vi "LAKESHORE_10_01_2023_R_VS_T_DEMO_1.vi"() -> ()   [LabVIEW 2020]
panel:
  out "Resistance":dbl
  out "Temperature":dbl
  in  "Channel":T1(ring)
  in  "VISA resource name":refnum<visa-resource-name>
  # "LAKE SHORE 372"
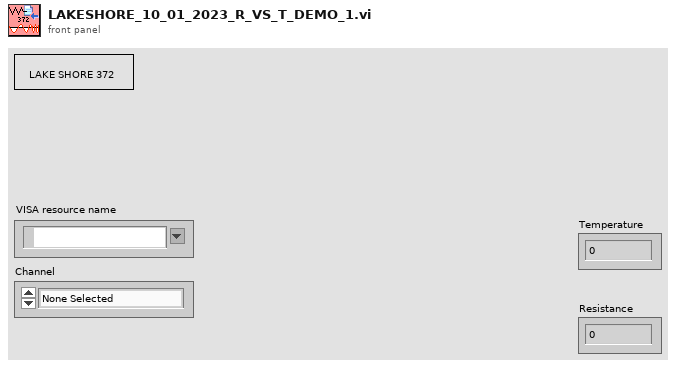
[diagram p1: front panel]
types:
  T1 = enum16{"None Selected", "1", "2", "3", "4", "5", "6", "7", "8", "9", "10", "11", "12", "13", "14", "15", "16"}
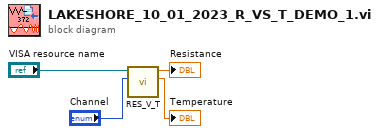
[diagram p0: block diagram]
diagram:
  n1 = call "RES_V_T.vi"("Channel"="Channel", "VISA Refnum in"="VISA resource name") -> ("Numeric 2"=→"Temperature":dbl, "Numeric"=→"Resistance":dbl)  [unwired: 8 in]
